vi "oa_Get Max Axis Display Value.vi"(7 "reset? (F)":bool, 8 "error in (no error)":errorcluster, 9 "orbit data Y":dbl[](array[numeric]), 10 "orbit data X":dbl[](array[numeric]), 11 "orbit plot ref":refnum<vi>) -> (0 "error out":errorcluster, 2 "max data value out":dbl, 3 "orbit plot out":refnum<vi>)   [LabVIEW 2017]
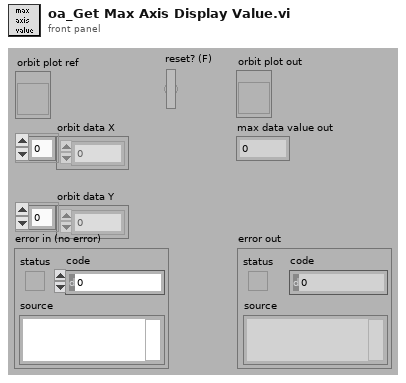
[diagram p1: front panel]
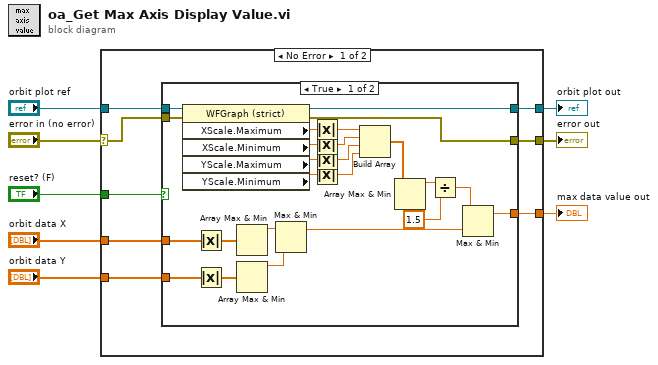
[diagram p0: block diagram]
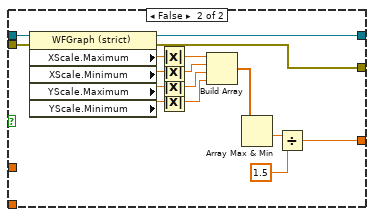
[diagram p2: hidden frame]
diagram:
  n1 = case shown="No Error" "error in (no error)" {
    selector: "error in (no error)" -> [w13 w57]
    tunnel: [w10 _] -> w8
    tunnel: "orbit data Y" -> [w16 _]
    tunnel: "orbit data X" -> [w15 _]
    tunnel: "orbit plot ref" -> [w14 w58]
    tunnel: [w12 w58] -> w3
    tunnel: [w11 w57] -> w2
    tunnel: "reset? (F)" -> [w9 _]
    frame No Error {
      n2 = case shown="True" w9 {
        tunnel: w16 -> [w36 _]
        tunnel: w15 -> [w35 _]
        tunnel: w14 -> [w34 w56]
        tunnel: w13 -> [w33 w55]
        tunnel: [w28 w50] -> w12
        tunnel: [w27 w49] -> w11
        tunnel: [w17 w42] -> w10
        frame True {
          n3 = property class="WFGraph (strict)"(reference=w34, error in=w33) -> (reference out=w28:refnum<vi>, error out=w27:errorcluster, "XScale.Maximum"=w32:dbl, "XScale.Minimum"=w31:dbl, "YScale.Maximum"=w30:dbl, "YScale.Minimum"=w29:dbl)
          n4 = Absolute Value(x=w35) -> (abs(x)=w39:dbl[])
          n5 = Absolute Value(x=w36) -> (abs(x)=w40:dbl[])
          n6 = Array Max & Min(array=w39) -> (max value=w37:dbl)  [unwired: 3 out]
          n7 = Array Max & Min(array=w40) -> (max value=w38:dbl)  [unwired: 3 out]
          n8 = Max & Min(x=w37, y=w38) -> (max(x,y)=w18:dbl)  [unwired: 1 out]
          n9 = Absolute Value(x=w32) -> (abs(x)=w26:dbl)
          n10 = Absolute Value(x=w31) -> (abs(x)=w25:dbl)
          n11 = Absolute Value(x=w30) -> (abs(x)=w24:dbl)
          n12 = Absolute Value(x=w29) -> (abs(x)=w23:dbl)
          n13 = Build Array(w26, w25, w24, w23) -> (w22:dbl[])
          n14 = Array Max & Min(array=w22) -> (max value=w21:dbl)  [unwired: 3 out]
          n15 = Divide(x=w21, y=1.5) -> (x/y=w20:dbl)
          n16 = Max & Min(x=w20, y=w18) -> (max(x,y)=w17:dbl)  [unwired: 1 out]
        }
        frame False {
          n17 = property class="WFGraph (strict)"(reference=w56, error in=w55) -> (reference out=w50:refnum<vi>, error out=w49:errorcluster, "XScale.Maximum"=w54:dbl, "XScale.Minimum"=w53:dbl, "YScale.Maximum"=w52:dbl, "YScale.Minimum"=w51:dbl)
          n18 = Absolute Value(x=w54) -> (abs(x)=w48:dbl)
          n19 = Absolute Value(x=w53) -> (abs(x)=w47:dbl)
          n20 = Absolute Value(x=w52) -> (abs(x)=w46:dbl)
          n21 = Absolute Value(x=w51) -> (abs(x)=w45:dbl)
          n22 = Build Array(w48, w47, w46, w45) -> (w44:dbl[])
          n23 = Array Max & Min(array=w44) -> (min value=w41:dbl)  [unwired: 3 out]
          n24 = Divide(x=w41, y=1.5) -> (x/y=w42:dbl)
        }
      }
    }
    frame Error {
    }
  }
  "max data value out" <- w8
  "orbit plot out" <- w3
  "error out" <- w2
